vi "DeppPutReg.vi"(7 "Overlap?":bool, 8 "Error In":errorcluster, 9 "Data":u8, 10 "Address":u8, 11 "Device Handle":u32) -> (0 "Error Out":errorcluster, 3 "Device Handle":u32)   [LabVIEW 2011, in "LVH-Adept.lvlib" / "DEPP.lvlib"]
uses:
  DEPP.lvlib
  Private/Type Defs/Error.ctl
  Resources/depp.dll
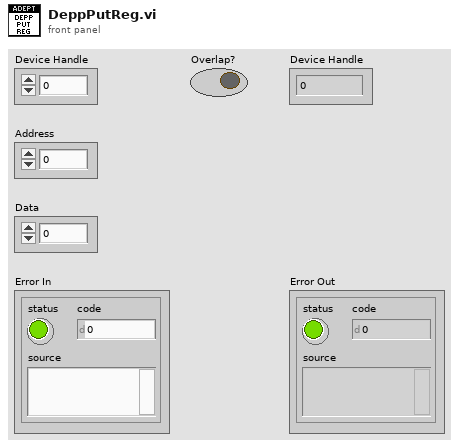
[diagram p1: front panel]
types:
  T1 = typedef "LVH-Adept.lvlib/DEPP.lvlib/Error.ctl" = enum16{"Unknown", "Enable", "Enable Port", "Get Register", "Get Register Repeat", "Get Register Set", "Put Register", "Put Register Repeat", "Put Register Set", "Disable", "Set Pair Size"}
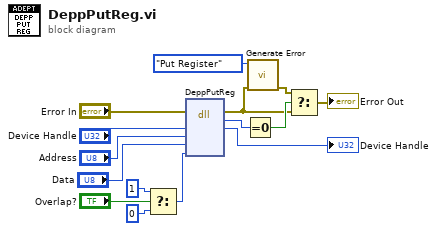
[diagram p0: block diagram]
diagram:
  n1 = Select(t=u8 1, s="Overlap?", f=u8 0) -> (s? t:f=w2:u8)
  n2 = dll-call lib="C:/github/labviewhacker/LVH-Adept/LabVIEW/vi.lib/LabVIEW Hacker/Adept/Private/Resources/depp.dll" fn="DeppPutReg"(error in="Error In", "hif"="Device Handle", "bAddr"="Address", "bData"="Data", "fOverlap"=w2) -> (error out=w7:errorcluster, "Success"=w14:u32, "hif"=→"Device Handle":u32)  [unwired: 5 in, 1 out]
  n3 = Equal To 0?(x=w14) -> (x = 0?=w13:bool)
  n4 = call "Generate Error.vi"("Error In"=w7, "DEPP Error"=Error."Put Register") -> ("Error Out"=w8:errorcluster)  [unwired: 9 in]
  n5 = Select(t=w8, s=w13, f=w7) -> (s? t:f=→"Error Out":errorcluster)
